vi "onStart.vi"(8 "error in (no error)":errorcluster, 11 "MQTT_Base in":refnum<class "MQTT_Base.lvclass">) -> (0 "error out":errorcluster, 3 "MQTT_Base out":refnum<class "MQTT_Base.lvclass">)   [LabVIEW 2013, in "MQTT Base.lvlib" / "MQTT_Base.lvclass"]
uses:
  MQTT_Base.lvclass
  MQTT_Base.lvclass/MQTT_Base.ctl
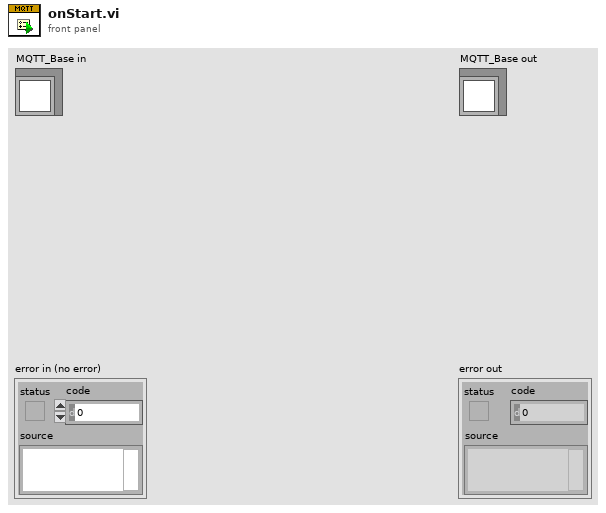
[diagram p1: front panel]
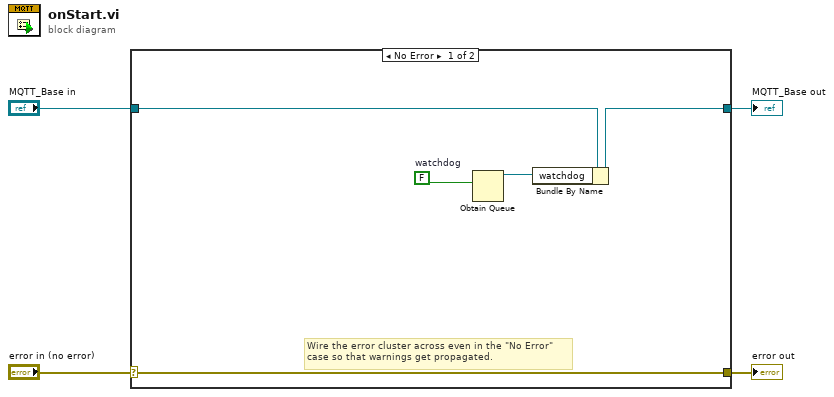
[diagram p0: block diagram]
diagram:
  n1 = case shown="No Error" "error in (no error)" {
    selector: "error in (no error)" -> [w9 w11]
    tunnel: [w9 w11] -> w3
    tunnel: [w7 w10] -> w1
    tunnel: "MQTT_Base in" -> [w8 w10]
    frame No Error {
      w5 = FALSE  # watchdog
      # "Wire the error cluster across even in the \"No Error\"\ncase so that warnings get propagated."
      n2 = Obtain Queue(element data type=w5) -> (queue out=w6:refnum<queue>)  [unwired: 4 in, 2 out]
      n3 = Bundle By Name(cluster=w8, "watchdog"=w6) -> (w7:refnum<class "MQTT_Base.lvclass">)
    }
    frame Error {
    }
  }
  "error out" <- w3
  "MQTT_Base out" <- w1
